vi "Untitled 1.vi"() -> ()   [LabVIEW 2015]
panel:
  out "channel name":string
  out "error out 4":errorcluster {"code" format="%.0x"}
  in  "instrument handle":refnum<k15>
  in  "channel index (1)":i32=1
  in  "error in (no error)":errorcluster {"code" format="%.0x"}
  out "instrument handle out":refnum<k15>
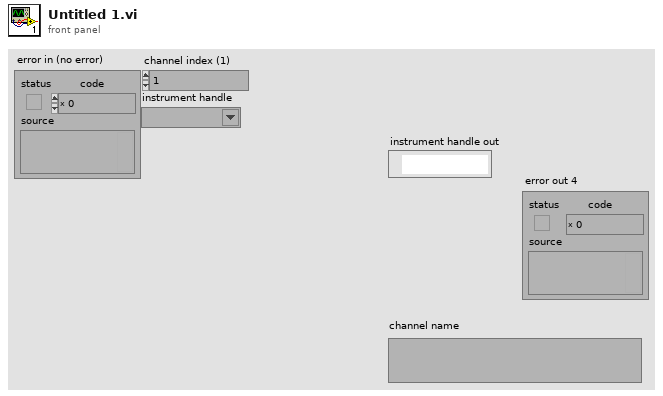
[diagram p1: front panel]
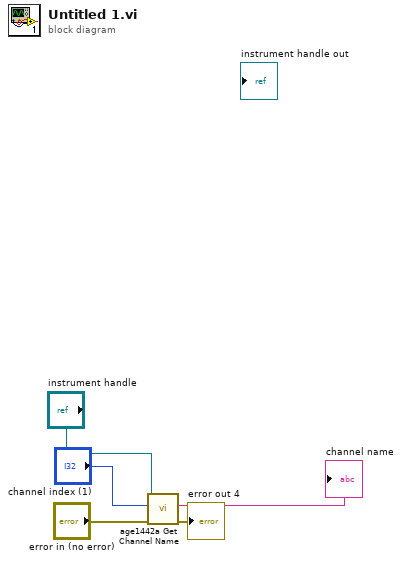
[diagram p0: block diagram]
diagram:
  n1 = call <instrlib>:"age1442a Get Channel Name.vi"("error in (no error)"="error in (no error)", "channel index (1)"="channel index (1)", "instrument handle"="instrument handle") -> ("error out"=→"error out 4":errorcluster, "channel name"=→"channel name":string)  [unwired: 6 in, 1 out]
